vi "Add Without Dup Priv.vi"(4 "Unique ID":string, 5 "Child IDs In":string[](array[string])) -> (2 "Child IDs Out":string[](array[string]))   [LabVIEW 2016, in "Tree Manager.lvclass"]
uses:
  Tree Manager.lvclass
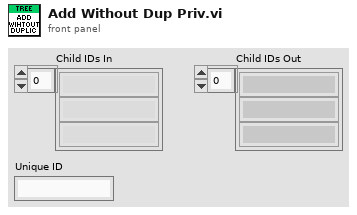
[diagram p1: front panel]
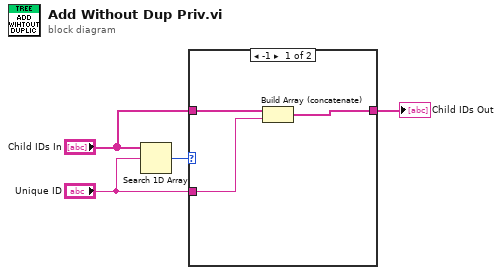
[diagram p0: block diagram]
diagram:
  n1 = Search 1D Array(1D array="Child IDs In", element="Unique ID") -> (index of element=w4:i32)  [unwired: 1 in]
  n2 = case shown="-1" w4 {
    tunnel: "Child IDs In" -> [w7 w8]
    tunnel: "Unique ID" -> [w6 _]
    tunnel: [w5 w8] -> w1
    frame -1 {
      n3 = Build Array (concatenate)(w7, w6) -> (w5:string[])
    }
    frame Default {
    }
  }
  "Child IDs Out" <- w1
